vi "Client Pool FGV.vi"(8 "error in (no error)":errorcluster, 11 "Action":T1) -> (0 "error out":errorcluster, 3 "grpc client id":T2)   [LabVIEW 2020, in "gRPC Utilities.lvlib" / "GrpcClientPool.lvclass"]
uses:
  GrpcClientPool.lvclass
  <vilib>/gRPC/LabVIEW gRPC Library/Shared/grpcId.ctl
  FGV Action.ctl
  <vilib>/gRPC/LabVIEW gRPC Library/grpc-lvsupport-release.lvlib
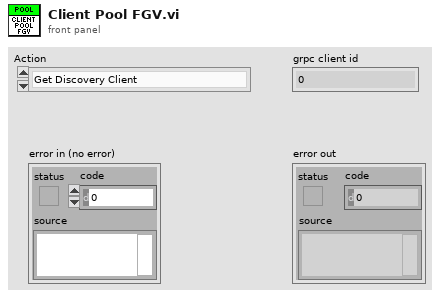
[diagram p1: front panel]
types:
  T1 = typedef "gRPC Utilities.lvlib/GrpcClientPool.lvclass/FGV Action.ctl" = enum16{"Get Discovery Client", "Get Session Client", "Get Pinmap Client", "Destroy Clients"}
  T2 = typedef "grpc-lvsupport-release.lvlib/grpcId.ctl" = u64
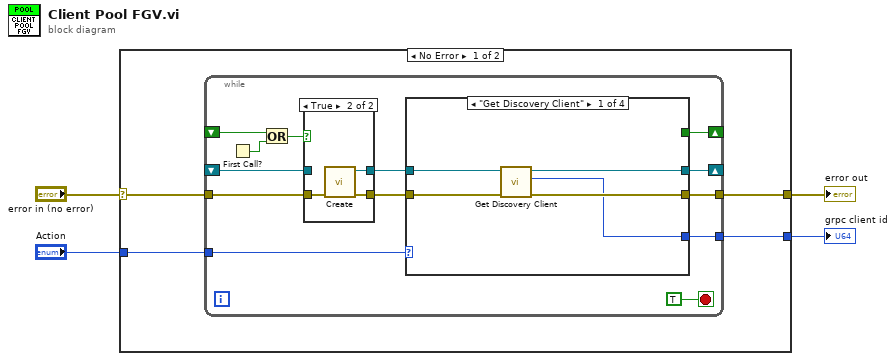
[diagram p0: block diagram]
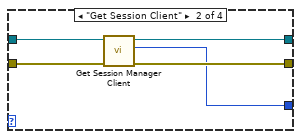
[diagram p3: hidden frame]
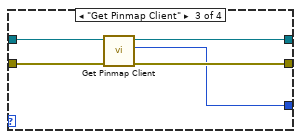
[diagram p4: hidden frame]
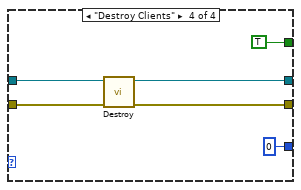
[diagram p5: hidden frame]
diagram:
  n1 = case shown="No Error" "error in (no error)" {
    selector: "error in (no error)" -> [w7 w48]
    tunnel: [w8 w48] -> w3
    tunnel: [w6 _] -> w2
    tunnel: "Action" -> [w5 _]
    frame No Error {
      n2 = while {
        tunnel: [w15] -> w8
        shift-right: [w17] -> _
        shift-left: _ -> [w19]
        tunnel: w7 -> [w20]
        tunnel: [w14] -> w6
        tunnel: w5 -> [w13]
        shift-right: [w12] -> _
        shift-left: _ -> [w9]
        stop <- TRUE stop-if-true
        n3 = First Call?() -> (First Call?: T/F=w11:bool)
        n4 = Or(x=w9, y=w11) -> (x .or. y?=w10:bool)
        n5 = case shown="True" w10 {
          tunnel: w20 -> [w23 w26]
          tunnel: [w23 w25] -> w16
          tunnel: [w22 w24] -> w18
          tunnel: w19 -> [w22 _]
          frame False {
          }
          frame True {
            n6 = call "Create.vi"("error in (no error)"=w26) -> ("error out"=w25:errorcluster, "ClientPool out"=w24:refnum<class "GrpcClientPool.lvclass">)  [unwired: 9 in]
          }
        }
        n7 = case shown="\"Get Discovery Client\"" w13 {
          tunnel: w18 -> [w30 w36 w41 w47]
          tunnel: [w29 w35 w40 w45] -> w17
          tunnel: w16 -> [w31 w34 w39 w46]
          tunnel: [w28 w33 w38 w44] -> w15
          tunnel: [w27 w32 w37 T2 0 ("Pinmap grpc id")] -> w14
          tunnel: [_ _ _ TRUE] -> w12
          frame "Get Discovery Client" {
            n8 = call "Get Discovery Client.vi"("error in (no error)"=w31, "ClientPool in"=w30) -> ("error out"=w28:errorcluster, "Discovery grpc id"=w27:T2, "ClientPool out"=w29:refnum<class "GrpcClientPool.lvclass">)  [unwired: 7 in]
          }
          frame "Get Session Client" {
            n9 = call "Get Session Manager Client.vi"("error in (no error)"=w34, "ClientPool in"=w36) -> ("error out"=w33:errorcluster, "Session manger grpc id"=w32:T2, "ClientPool out"=w35:refnum<class "GrpcClientPool.lvclass">)  [unwired: 7 in]
          }
          frame "Get Pinmap Client" {
            n10 = call "Get Pinmap Client.vi"("error in (no error)"=w39, "ClientPool in"=w41) -> ("error out"=w38:errorcluster, "Pinmap grpc id"=w37:T2, "ClientPool out"=w40:refnum<class "GrpcClientPool.lvclass">)  [unwired: 7 in]
          }
          frame "Destroy Clients" {
            n11 = call "Destroy.vi"("error in (no error)"=w46, "ClientPool in"=w47) -> ("error out"=w44:errorcluster, "ClientPool out"=w45:refnum<class "GrpcClientPool.lvclass">)  [unwired: 8 in]
          }
        }
      }
    }
    frame Error {
    }
  }
  "error out" <- w3
  "grpc client id" <- w2
